vi "Power_spectrumOld.vi"(0 "U":dbl[](array[numeric]) format="%.2f", 2 "Sampling frequency":sgl format="%.2f", 3 "Spectrum input array":dbl[](array[numeric]) format="%.2f", 4 "Block No":i32=1) -> (6 "Spectrum output array":dbl[](array[numeric]) format="%.2f")   [LabVIEW 2012]
uses:
  <vilib>/Analysis/baseanly.llb/Mean (DBL).vi
  <vilib>/Analysis/2dsp.llb/Power Spectrum (DBL).vi
  <vilib>/Analysis/NI_AALPro.lvlib
  <vilib>/Analysis/NI_AALBase.lvlib
panel:
  out "size(s)":i32
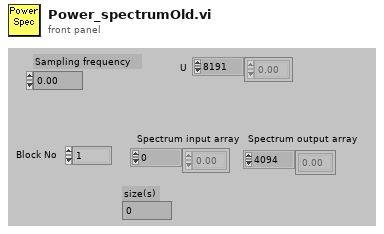
[diagram p1: front panel]
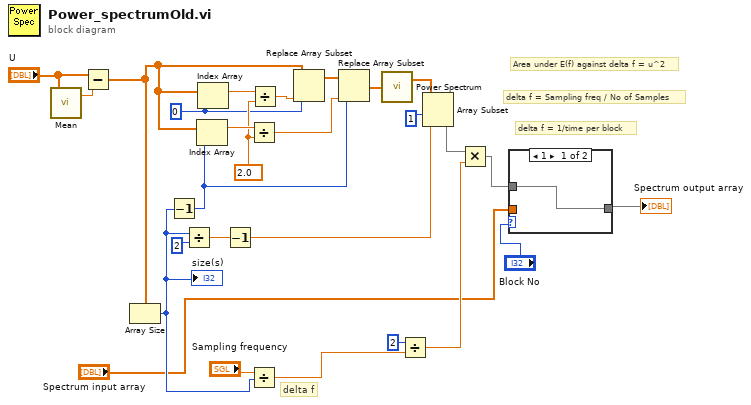
[diagram p0: block diagram]
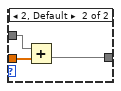
[diagram p2: hidden frame]
diagram:
  w21 = 2.0
  w20 = 0
  # "delta f"
  # "Area under E(f) against delta f = u^2"
  # "delta f = 1/time per block"
  # "delta f = Sampling freq / No of Samples"
  n1 = call-poly <vilib>:"Mean.vi"("X"="U") -> ("mean"=w13:dbl)  [unwired: 1 out]
  n2 = Subtract(x="U", y=w13) -> (x-y=w3:dbl[])
  n3 = Array Size(array=w3) -> (size(s)=w12:i32)
  "size(s)" <- w12
  n4 = Decrement(x=w12) -> (x-1=w17:i32)
  n5 = Divide(x=w12, y=2) -> (x/y=w5:dbl)
  n6 = Index Array(array=w3, index=w17) -> (element=w22:dbl)
  n7 = Index Array(array=w3, index=w20) -> (element=w23:dbl)
  n8 = Decrement(x=w5) -> (x-1=w4:dbl)
  n9 = Divide(x=w22, y=w21) -> (x/y=w18:dbl)
  n10 = Divide(x="Sampling frequency", y=w12) -> (x/y=w9:sgl)
  n11 = Divide(x=w23, y=w21) -> (x/y=w19:dbl)
  n12 = Replace Array Subset(array=w3, new element=w19, index=w20) -> (w24:dbl[])
  n13 = Replace Array Subset(array=w24, new element=w18, index=w17) -> (w16:dbl[])
  n14 = call-poly <vilib>:"Power Spectrum.vi"("X"=w16) -> ("Power Spectrum"=w25:dbl[])  [unwired: 1 out]
  n15 = Divide(x=2, y=w9) -> (x/y=w11:sgl)
  n16 = Array Subset(array=w25, index=1, length=w4) -> (w10:dbl[])
  n17 = Multiply(x=w10, y=w11) -> (x*y=w1:dbl[])
  n18 = case shown="1" "Block No" {
    tunnel: [w28 w31] -> w2
    tunnel: w1 -> [w28 w30]
    tunnel: "Spectrum input array" -> [_ w29]
    frame 1 {
    }
    frame 2, Default {
      n19 = Add(x=w30, y=w29) -> (x+y=w31:dbl[])
    }
  }
  "Spectrum output array" <- w2
